vi "Servo Button.vi"() -> ()   [LabVIEW 2013]
panel:
  in  "Shoot Button":bool
  in  "Override Shoot":bool
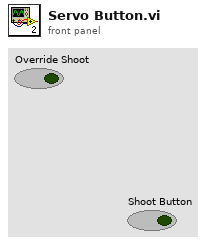
[diagram p1: front panel]
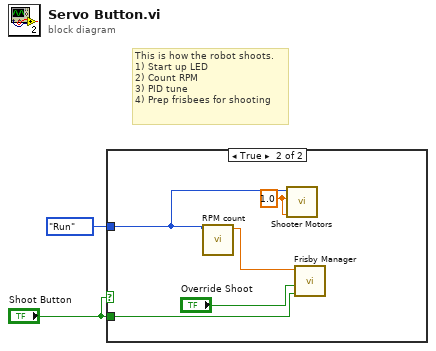
[diagram p0: block diagram]
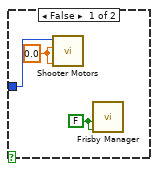
[diagram p2: hidden frame]
diagram:
  # "This is how the robot shoots.\n1) Start up LED\n2) Count RPM\n3) PID tune\n4) Prep frisbees for shooting"
  n1 = case shown="True" "Shoot Button" {
    tunnel: enum16{"Open", "Run", "End"}."Run" ("State Control") -> [w4 w7]
    tunnel: "Shoot Button" -> [_ w9]
    frame False {
      w3 = FALSE ("Override Shoot")
      w5 = 0.0 ("Front Shooter Motor")
      n2 = call "Shooter Motors.vi"("Back Shooter Motor"=w5, "Front Shooter Motor"=w5, "State Control"=w4) -> ()  [unwired: 9 in]
      n3 = call "Frisby Manager.vi"("I wanna shoot"=w3, "Override Shoot"=w3) -> ()  [unwired: 10 in]
    }
    frame True {
      w6 = 1.0 ("Front Shooter Motor")
      n4 = call "RPM count.vi"("State Control"=w7) -> ("RPM"=w8:dbl)  [unwired: 10 in]
      n5 = call "Shooter Motors.vi"("Back Shooter Motor"=w6, "Front Shooter Motor"=w6, "State Control"=w7) -> ()  [unwired: 9 in]
      n6 = call "Frisby Manager.vi"("I wanna shoot"=w9, "Override Shoot"="Override Shoot", "Current RPM"=w8) -> ()  [unwired: 9 in]
    }
  }
